vi "Servo.vi"(7 "Action":T1, 8 "error in (no error)":errorcluster, 10 "Angle (deg)":i32, 11 "ServoDeviceRef":T2={"DeviceStatus"={"status"=FALSE, "code"=0, "source"=""}, "Digital Module"=enum."Digital Module 1", "PWM Channel"=enum."Invalid", "DeadBand"={"Name"="", "maxPositivePwm"=0, "minPositivePwm"=0, "centerPwm"=0, "maxNegativePwm"=0, "minNegativePwm"=0, "angularRange"=0}}) -> (0 "error out":errorcluster, 2 "Angle (deg)":i32)   [LabVIEW 2015]
doc: "VI for controlling the servo. It has the following actions:\n-Init: takes a servo reference and stores it.\n-GetAngle: returns the current angle of the servo.\n-SetAngle: sets the servo to the specified angle.\n-Raise: increases the servo angle by 1.\n-Lower: decreases the servo angle by 1, but never sets the angle past 0.\n-Disable: no action, except for reporting the current angle to the dashboard."
uses:
  <vilib>/Rock Robotics/WPI/PWM/Servo/WPI_ServoDeviceRef.ctl
  <vilib>/Rock Robotics/SystemInterfaces/Typedef/FPGA_TypedefDigitalModule.ctl
  <vilib>/Rock Robotics/SystemInterfaces/DIO/FPGA_DIOPWMChannel.ctl
  <vilib>/Rock Robotics/WPI/PWM/WPI_PWMDeadband.ctl
  ServoAction.ctl
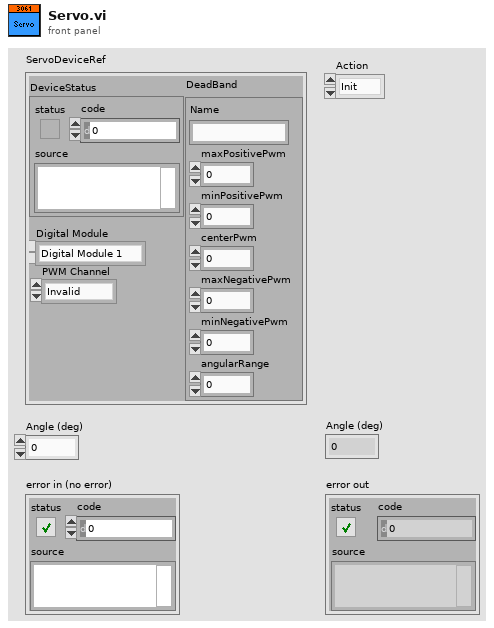
[diagram p1: front panel]
types:
  T1 = typedef "ServoAction.ctl" = enum16{"Init", "SetAngle", "GetAngle", "Lower", "Raise", "Disable"}
  T2 = typedef "WPI_ServoDeviceRef.ctl" = cluster{"DeviceStatus":errorcluster, "Digital Module":T3, "PWM Channel":T4, "DeadBand":T5}
  T3 = typedef "FPGA_TypedefDigitalModule.ctl" = enum16{"Digital Module 1", "Digital Module 2"}
  T4 = typedef "FPGA_DIOPWMChannel.ctl" = enum8{"PWM 1", "PWM 2", "PWM 3", "PWM 4", "PWM 5", "PWM 6", "PWM 7", "PWM 8", "PWM 9", "PWM 10", "Invalid"}
  T5 = typedef "WPI_PWMDeadband.ctl" = cluster{"Name":string, "maxPositivePwm":i32, "minPositivePwm":i32, "centerPwm":i32, "maxNegativePwm":i32, "minNegativePwm":i32, "angularRange":u16}
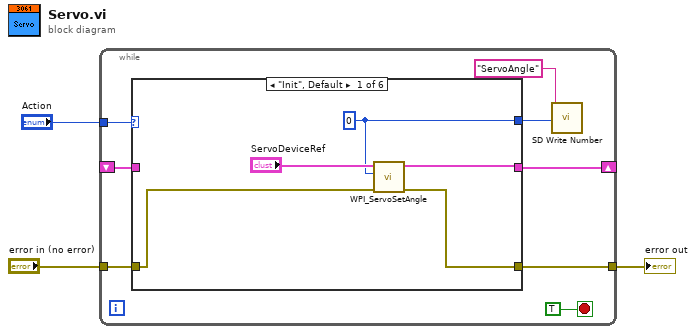
[diagram p0: block diagram]
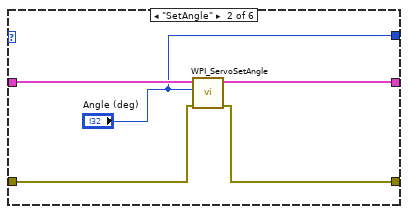
[diagram p2: hidden frame]
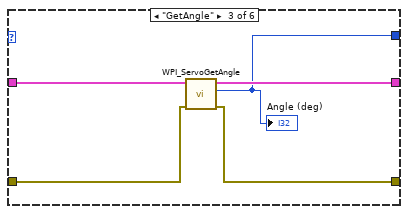
[diagram p3: hidden frame]
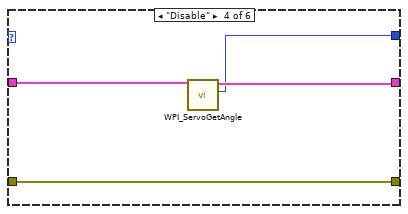
[diagram p4: hidden frame]
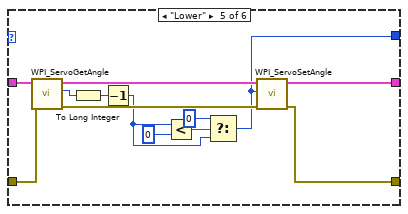
[diagram p5: hidden frame]
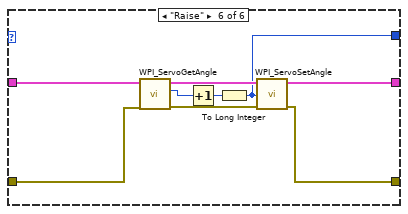
[diagram p6: hidden frame]
diagram:
  n1 = while {
    tunnel: "Action" -> [w10]
    shift-right: [w9] -> _
    shift-left: _ -> [w8]
    tunnel: "error in (no error)" -> [w7]
    tunnel: [w6] -> w1
    stop <- TRUE stop-if-true
    n2 = case shown="\"Init\", Default" w10 {
      tunnel: [w15 w20 w25 w29 w40 w50] -> w9
      tunnel: w8 -> [_ w21 w26 w30 w41 w52]
      tunnel: w7 -> [w14 w19 w24 w27 w39 w46]
      tunnel: [w13 w18 w23 w27 w38 w47] -> w6
      tunnel: [w12 "Angle (deg)" w22 w28 w33 w44] -> w5
      frame "Init", Default {
        w12 = 0 ("Angle (deg)")
        n3 = call <vilib>:"WPI_ServoSetAngle.vi"("error in (no error)"=w14, "Angle"=w12, "ServoDeviceRef"="ServoDeviceRef") -> ("error out"=w13:errorcluster, "ServoDeviceRef"=w15:T2)  [unwired: 7 in]
      }
      frame "SetAngle" {
        n4 = call <vilib>:"WPI_ServoSetAngle.vi"("error in (no error)"=w19, "Angle"="Angle (deg)", "ServoDeviceRef"=w21) -> ("error out"=w18:errorcluster, "ServoDeviceRef"=w20:T2)  [unwired: 7 in]
      }
      frame "GetAngle" {
        n5 = call <vilib>:"WPI_ServoGetAngle.vi"("ServoDeviceRef"=w26, "error in (no error)"=w24) -> ("ServoDeviceRef"=w25:T2, "Angle"=w22:u16, "error out"=w23:errorcluster)  [unwired: 6 in]
        "Angle (deg)" <- w22
      }
      frame "Disable" {
        n6 = call <vilib>:"WPI_ServoGetAngle.vi"("ServoDeviceRef"=w30) -> ("ServoDeviceRef"=w29:T2, "Angle"=w28:u16)  [unwired: 7 in, 1 out]
      }
      frame "Lower" {
        n7 = call <vilib>:"WPI_ServoGetAngle.vi"("ServoDeviceRef"=w41, "error in (no error)"=w39) -> ("ServoDeviceRef"=w43:T2, "Angle"=w32:u16, "error out"=w42:errorcluster)  [unwired: 6 in]
        n8 = To Long Integer(number=w32) -> (32bit integer=w34:i32)
        n9 = Decrement(x=w34) -> (x-1=w31:i32)
        n10 = Less?(x=w31, y=0) -> (x < y?=w36:bool)
        n11 = Select(t=0 ("y"), s=w36, f=w31) -> (s? t:f=w33:i32)
        n12 = call <vilib>:"WPI_ServoSetAngle.vi"("error in (no error)"=w42, "Angle"=w33, "ServoDeviceRef"=w43) -> ("error out"=w38:errorcluster, "ServoDeviceRef"=w40:T2)  [unwired: 7 in]
      }
      frame "Raise" {
        n13 = call <vilib>:"WPI_ServoGetAngle.vi"("ServoDeviceRef"=w52, "error in (no error)"=w46) -> ("ServoDeviceRef"=w51:T2, "Angle"=w49:u16, "error out"=w48:errorcluster)  [unwired: 6 in]
        n14 = Increment(x=w49) -> (x+1=w45:u16)
        n15 = To Long Integer(number=w45) -> (32bit integer=w44:i32)
        n16 = call <vilib>:"WPI_ServoSetAngle.vi"("error in (no error)"=w48, "Angle"=w44, "ServoDeviceRef"=w51) -> ("error out"=w47:errorcluster, "ServoDeviceRef"=w50:T2)  [unwired: 7 in]
      }
    }
    n17 = call <vilib>:"SD Write Number.vi"("Numeric"=w5, "Name"="ServoAngle") -> ()  [unwired: 8 in, 2 out]
  }
  "error out" <- w1
